vi "recipeScript getInstrCurrnetScript.vi"(8 "error in (no error)":errorcluster, 11 "Network\nstream":refnum<vi>) -> (0 "error out":errorcluster, 1 "versionInfo":string, 2 "initScriptCode":string, 3 "initFilePath":path, 5 "userParam":string)   [LabVIEW 2018]
uses:
  getScriptInfo.ctl
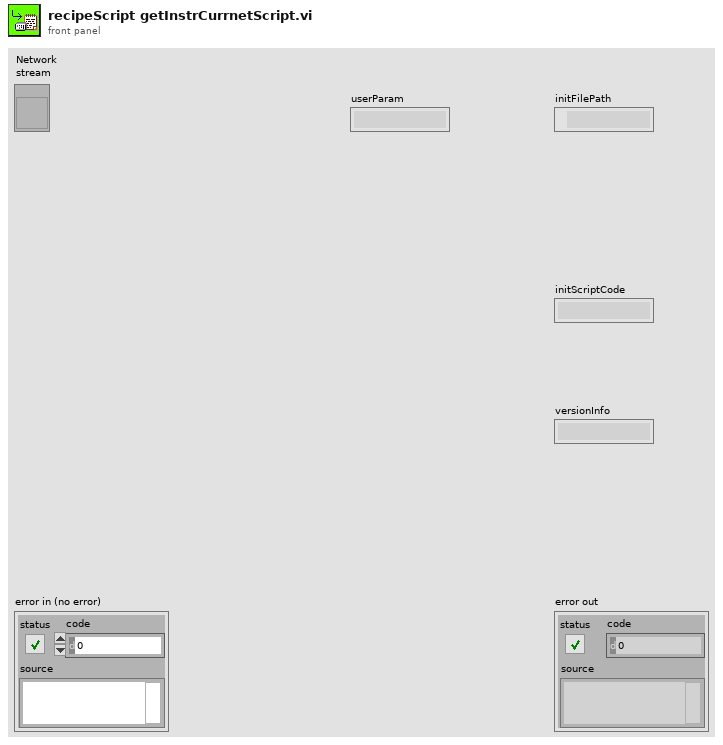
[diagram p1: front panel]
types:
  T1 = typedef "getScriptInfo.ctl" = enum16{"userEditor", "userParam", "instrParam", "sourcePath", "sourceTimeStamp", "versionInfo"}
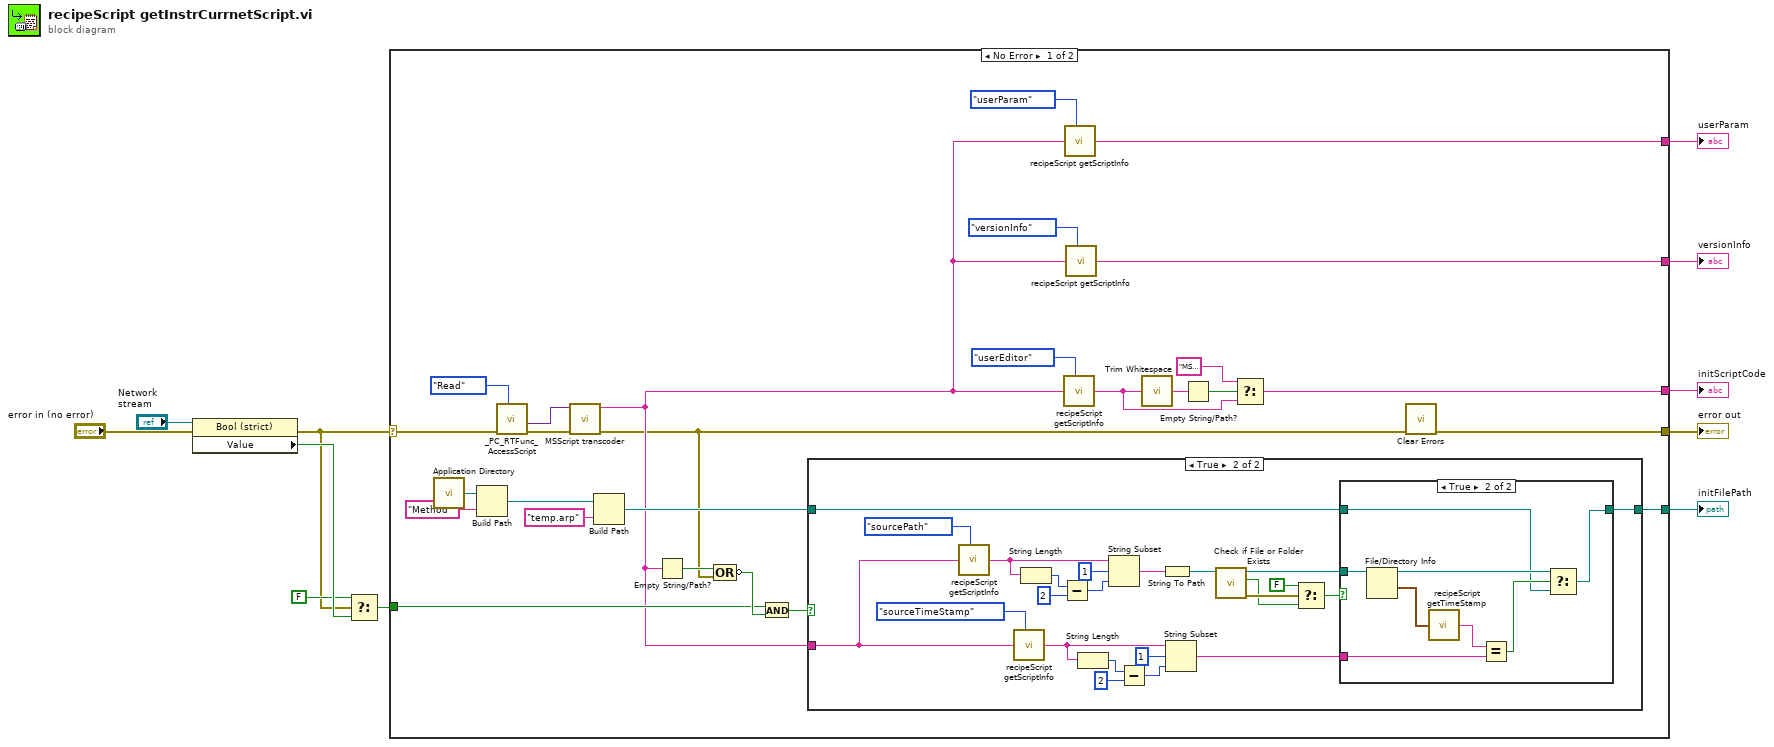
[diagram p0: block diagram]
diagram:
  n1 = property class="Bool (strict)"(reference="Network\nstream", error in="error in (no error)") -> (error out=w4:errorcluster, "Value"=w9:bool)  [unwired: 1 out]
  n2 = Select(t=FALSE, s=w4, f=w9) -> (s? t:f=w7:bool)
  n3 = case shown="No Error" w4 {
    selector: w4 -> [w28 w72]
    tunnel: [w23 _] -> w11
    tunnel: w7 -> [w27 _]
    tunnel: [w13 w72] -> w5
    tunnel: [w18 _] -> w3
    tunnel: [w14 _] -> w2
    tunnel: [w15 _] -> w1
    frame No Error {
      n4 = call <vilib>:"Application Directory.vi"() -> ("Application Directory"=w32:path)
      n5 = Build Path(base path=w32, name or relative path="Method") -> (appended path=w30:path)
      n6 = call "_PC_RTFunc_AccessScript.vi"("Function"=enum16{"Write", "Read"}."Read", "error in (no error)"=w28) -> ("error out"=w36:errorcluster, "Var out"=w37:variant)  [unwired: 8 in]
      n7 = call "MSScript transcoder.vi"("error in (no error)"=w36, "new value"=w37) -> ("error out"=w12:errorcluster, "script code"=w16:string)  [unwired: 8 in]
      n8 = Build Path(base path=w30, name or relative path="temp.arp") -> (appended path=w26:path)
      n9 = Empty String/Path?(string/path=w16) -> (empty?=w35:bool)
      n10 = Compound Arithmetic op=OR(w35, w12) -> (invert w34:bool)
      n11 = And(x=w27, y=w34) -> (x .and. y?=w33:bool)
      n12 = case shown="True" w33 {
        tunnel: w16 -> [_ w40]
        tunnel: w26 -> [w39 w48]
        tunnel: [w39 w47] -> w23
        frame False {
        }
        frame True {
          n13 = call "recipeScript getScriptInfo.vi"("sysCode"=w40, "method"=getScriptInfo."sourcePath") -> ("output"=w61:string)  [unwired: 1 in]
          n14 = call "recipeScript getScriptInfo.vi"("sysCode"=w40, "method"=getScriptInfo."sourceTimeStamp") -> ("output"=w51:string)  [unwired: 1 in]
          n15 = String Length(string=w61) -> (length=w60:i32)
          n16 = Subtract(x=w60, y=2) -> (x-y=w58:i32)
          n17 = String Length(string=w51) -> (length=w54:i32)
          n18 = String Subset(string=w61, offset (0)=1, length (rest)=w58) -> (substring=w57:string)
          n19 = Subtract(x=w54, y=2) -> (x-y=w52:i32)
          n20 = String To Path(string=w57) -> (path=w56:path)
          n21 = String Subset(string=w51, offset (0)=1, length (rest)=w52) -> (substring=w49:string)
          n22 = call <vilib>:"Check if File or Folder Exists.vi"("path"=w56) -> ("error out"=w46:errorcluster, "file or folder exists?"=w45:bool, "dup path"=w50:path)  [unwired: 8 in]
          n23 = Select(t=FALSE, s=w46, f=w45) -> (s? t:f=w43:bool)
          n24 = case shown="True" w43 {
            tunnel: w50 -> [_ w71]
            tunnel: w49 -> [_ w70]
            tunnel: w48 -> [w63 w67]
            tunnel: [w63 w66] -> w47
            frame False {
            }
            frame True {
              n25 = File/Directory Info(path=w71) -> (path out=w68:path, last mod=w65:timestamp)  [unwired: 1 in, 5 out]
              n26 = call "recipeScript getTimeStamp.vi"("timeFormat"=w65) -> ("timeStamp"=w64:string)
              n27 = Equal?(x=w64, y=w70) -> (x = y?=w69:bool)
              n28 = Select(t=w68, s=w69, f=w67) -> (s? t:f=w66:path)
            }
          }
        }
      }
      n29 = call "recipeScript getScriptInfo.vi"("sysCode"=w16, "method"=getScriptInfo."userEditor") -> ("output"=w19:string)  [unwired: 1 in]
      n30 = call "recipeScript getScriptInfo.vi"("sysCode"=w16, "method"=getScriptInfo."userParam") -> ("output"=w15:string)  [unwired: 1 in]
      n31 = call "recipeScript getScriptInfo.vi"("sysCode"=w16, "method"=getScriptInfo."versionInfo") -> ("output"=w14:string)  [unwired: 1 in]
      n32 = call <vilib>:"Trim Whitespace.vi"("string"=w19) -> ("trimmed string"=w22:string)  [unwired: 1 in]
      n33 = Empty String/Path?(string/path=w22) -> (empty?=w21:bool)
      n34 = Select(t="MSProcess.Header( 10, 7.07107, 330 );\n\nMSProcess.UpdConj( 2147483648, [0,0], [2147483648,2147483648], F );\n\nMSProcess.SetDAQ( 1, 0 );\n\nMSProcess.UpdDO( [1,0,0,0], [F,F,F,F] );\nMSProcess.UpdAO( [0,0,0,0], [-3,0,0,0] );\n\nMSProcess.UpdRFChFunc( 1, 1, 1 );\nMSProcess.UpdRFChBias( 0, 0, 0 );\nMSProcess.UpdRFChScale( 1, 1, 1 );\nMSProcess.UpdConj( 2147483648, [0,0], [2147483648,2147483648], F );\n\nMSProcess.RFStart( 300000, 200, 0 );\n\nMSProcess.PhaseScan( 2, 0, 0, 2, 1, 1, 0, [0.2,0.25], [0.4,0.45], [-0.2,0], 0.1, [300000,200000], 5 )\n\nMSProcess.RFStop();" ("Text"), s=w21, f=w19) -> (s? t:f=w18:string)
      n35 = call <vilib>:"Clear Errors.vi"("error in (no error)"=w12) -> ("error out"=w13:errorcluster)  [unwired: 5 in, 1 out]
    }
    frame Error {
    }
  }
  "initFilePath" <- w11
  "initScriptCode" <- w3
  "error out" <- w5
  "versionInfo" <- w2
  "userParam" <- w1
